vi "Loop_SM.vi"() -> ()   [LabVIEW 2017, in "Claw_Rotation.lvlib"]
uses:
  Claw_Rotation.lvlib
  CLUSTER_CMD_SM_Lift_Rotate.ctl
  ENUM_SM_Rotate_Positions.ctl
  _SHARE ALL/TypeDef Share All/CLUSTER_TalonInput.ctl
  System Drivers/Phoenix-LabVIEW/Motor Controller/Controls/CTRE_Phoenix_MotorControl_ControlMode.ctl
  TypeDef/CLUSTER_PID.ctl
  ENUM_SM_State.ctl
  CLUSTER_ACT_Lift Output.ctl
  _SHARE ALL/RoboRio Share All/SRX Share All/TypeDefs SRX/Cluster_SRX_General Data.ctl
  _SHARE ALL/RoboRio Share All/SRX Share All/TypeDefs SRX/Cluster_SRX_Common Runtime Data.ctl
  _SHARE ALL/RoboRio Share All/SRX Share All/TypeDefs SRX/Cluster_SRX_Error Calculations.ctl
  _SHARE ALL/RoboRio Share All/SRX Share All/TypeDefs SRX/Cluster_SRX_Voltage Out Data.ctl
  _SHARE ALL/RoboRio Share All/SRX Share All/TypeDefs SRX/Cluster_SRX_Sensor Out Data.ctl
  _SHARE ALL/RoboRio Share All/SRX Share All/TypeDefs SRX/Cluster_SRX_Sensor Quad Data.ctl
  _SHARE ALL/RoboRio Share All/SRX Share All/TypeDefs SRX/Cluster_SRX_Analog In Data.ctl
  _SHARE ALL/RoboRio Share All/SRX Share All/TypeDefs SRX/Cluster_SRX_PWM Sensor Data.ctl
  _SHARE ALL/RoboRio Share All/SRX Share All/TypeDefs SRX/Cluster_SRX_F and R Limit Indicators.ctl
  ENUM_SM_Action.ctl
  Globals/Global_Device_IDs.vi
  _SHARE ALL/Global Share All/Global_STOP.vi
  Global_ACT Write_Data Out.vi
  Global_SM Write_Data Out.vi
  Global_CMD.vi
panel:
  in  "CMD_SM_Claw_Rotation":T1={"Enable System"=TRUE, "Rotate Position"=enum."Neutral: 0", "Manual Velocity"=0.0, "Manual Mode"=FALSE}
  out "State":T3
  out "SM Output":T4 {"Talon Mode" items=["PercentOutput"=0, "Position"=1, "Velocity"=2, "Current"=3, "Follower"=5, "MotionProfile"=6, "MotionMagic"=7, "MotionMagicArc"=8, "MotionProfileArc"=10, "Disabled"=15]}
  out "SM CMD Input":T1={"Enable System"=TRUE, "Rotate Position"=enum."Neutral: 0", "Manual Velocity"=0.0, "Manual Mode"=FALSE}
  out "Cycle Time (S)":dbl format="%.3g"
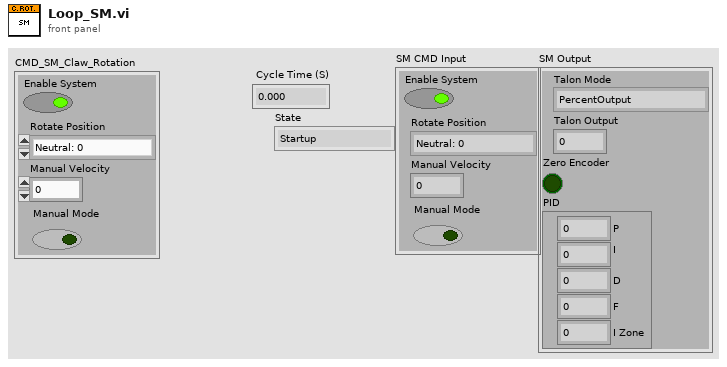
[diagram p1: front panel]
types:
  T1 = typedef "Claw_Rotation.lvlib/CLUSTER_CMD_SM_Lift_Rotate.ctl" = cluster{"Enable System":bool, "Rotate Position":T2, "Manual Velocity":dbl, "Manual Mode":bool}
  T2 = typedef "Claw_Rotation.lvlib/ENUM_SM_Rotate_Positions.ctl" = enum16{"Neutral: 0", "Pickup: 0", "Exchange: 0", "Switch: 0", "Scale: 0", "Climb: 0"}
  T3 = typedef "Claw_Rotation.lvlib/ENUM_SM_State.ctl" = enum16{"Startup", "Idle", "Manual", "Position - Moving", "Position - Holding", "Shutdown"}
  T4 = typedef "CLUSTER_TalonInput.ctl" = cluster{"Talon Mode":T5, "Talon Output":dbl, "Zero Encoder":bool, "PID":T6}
  T5 = typedef "CTRE_Phoenix_MotorControl_ControlMode.ctl" = u16
  T6 = typedef "CLUSTER_PID.ctl" = cluster{"P":dbl, "I":dbl, "D":dbl, "F":dbl, "I Zone":dbl}
  T7 = typedef "Claw_Rotation.lvlib/CLUSTER_ACT_Lift Output.ctl" = cluster{"Device Info Out":T8, "Common Runtime Data Out":T9, "Quad Sensor Data Out":T13, "Analog Sensor Data Out":T14, "PWM Data Out":T15, "Hard Limits Out":T16}
  T8 = typedef "Cluster_SRX_General Data.ctl" = cluster{"Device ID":i32, "Firmware Version":i32, "Inverted?":bool, "Has Reset Occurred?":bool}
  T9 = typedef "Cluster_SRX_Common Runtime Data.ctl" = cluster{"Calc":T10, "Voltage ":T11, "Sensor":T12, "Current":dbl, "Temp":dbl}
  T10 = typedef "Cluster_SRX_Error Calculations.ctl" = cluster{"Error":i32, "D-Error":dbl, "I-Acc":dbl}
  T11 = typedef "Cluster_SRX_Voltage Out Data.ctl" = cluster{"Percent":dbl, "Output":dbl, "Bus":dbl}
  T12 = typedef "Cluster_SRX_Sensor Out Data.ctl" = cluster{"Pos":i32, "Vel":i32}
  T13 = typedef "Cluster_SRX_Sensor Quad Data.ctl" = cluster{"Position":i32, "Velocity":i32, "Quad A Pin":bool, "Quad B Pin":bool, "Quad Idx Pin":bool}
  T14 = typedef "Cluster_SRX_Analog In Data.ctl" = cluster{"WithOv":i32, "Raw":i32, "Velocity":i32}
  T15 = typedef "Cluster_SRX_PWM Sensor Data.ctl" = cluster{"Position":i32, "Velocity":i32, "High(us)":i32, "Period(us)":i32}
  T16 = typedef "Cluster_SRX_F and R Limit Indicators.ctl" = cluster{"Forward Closed?":bool, "Reverse Closed?":bool}
  T17 = typedef "Claw_Rotation.lvlib/ENUM_SM_Action.ctl" = enum16{"No Action", "Reset Time", "Reset All", "Reset Encoder", "Manual", "Position", "Set PID 1", "Disable Motor"}
  T18 = typedef "CLUSTER_Talon_Setup.ctl" = cluster{"Open Data":T19, "Current Config Data":T20, "Sensor Config":T21, "Hard Limits":T23, "Motion Magic Config Data":T25, "PIDF":T26, "Maximum Integral Accumulator Value":dbl, "AllowableClosedLoop":i32, "Limits":T27, "Output Config":T28}
  T19 = typedef "Cluster_SRX_OPEN Data.ctl" = cluster{"SRX ID":u8, "Invert Output":bool}
  T20 = typedef "Cluster_SRX_Current Config.ctl" = cluster{"Enable Current Limit?":bool, "Peak Current (Amps)":i32, "Peak Current Maximum Duration (ms)":i32, "Continuous Current Limit (Amps)":i32}
  T21 = typedef "Cluster_SRX_Sensor Config.ctl" = cluster{"Feedback Device":T22, "PhaseSensor":bool}
  T22 = typedef "CTRE_Phoenix_MotorControl_FeedbackDevice.ctl" = i8
  T23 = typedef "Cluster_SRX_Config Hard Limits.ctl" = cluster{"Fwd Enable":bool, "Rev Enable":bool, "Fwd NO-NC":T24, "Rev NO-NC":T24}
  T24 = typedef "CTRE_Phoenix_MotorControl_LimitSwitchNormal.ctl" = enum16{"Normally Open", "Normally Closed", "Disabled"}
  T25 = typedef "Cluster_SRX_Motion Magic Config Data.ctl" = cluster{"Cruise Velocity":i32, "Acceleration":i32}
  T26 = typedef "Cluster_SRX_PIDF.ctl" = cluster{"P":dbl, "I":dbl, "D":dbl, "F":dbl, "I Zone":dbl}
  T27 = typedef "Cluster_SRX_Config Soft Limits.ctl" = cluster{"Max":i32, "Min":i32, "Max Enable":bool, "Min Enable":bool}
  T28 = typedef "Cluster_SRX_Config Voltage Output.ctl" = cluster{"Invert?":bool, "Neutral Mode":T29, "Deadband (-1to1)":dbl, "Ramp Time Off to Full (S)":dbl, "Peak  (-1to1)":T30, "Nominal  (-1to1)":T30}
  T29 = typedef "CTRE_Phoenix_MotorControl_NeutralMode.ctl" = enum8{"EEPROMSetting", "Override to Coast", "Override to Brake"}
  T30 = typedef "Cluster_SRX_Forward and Reverse.ctl" = cluster{"Forward":dbl, "Reverse":dbl}
  T31 = cluster{"State":T3, "Previous State":T3, "Current Time":timestamp, "Previous Time":timestamp, "Start Time":timestamp, "Target Time (ms)":u32, "Cycle Time(S)":dbl, "Claw_Rotation_Output":T7, "SM CMD Input":T1, "SM Output":T4, "Claw Rotation Setup":T18}
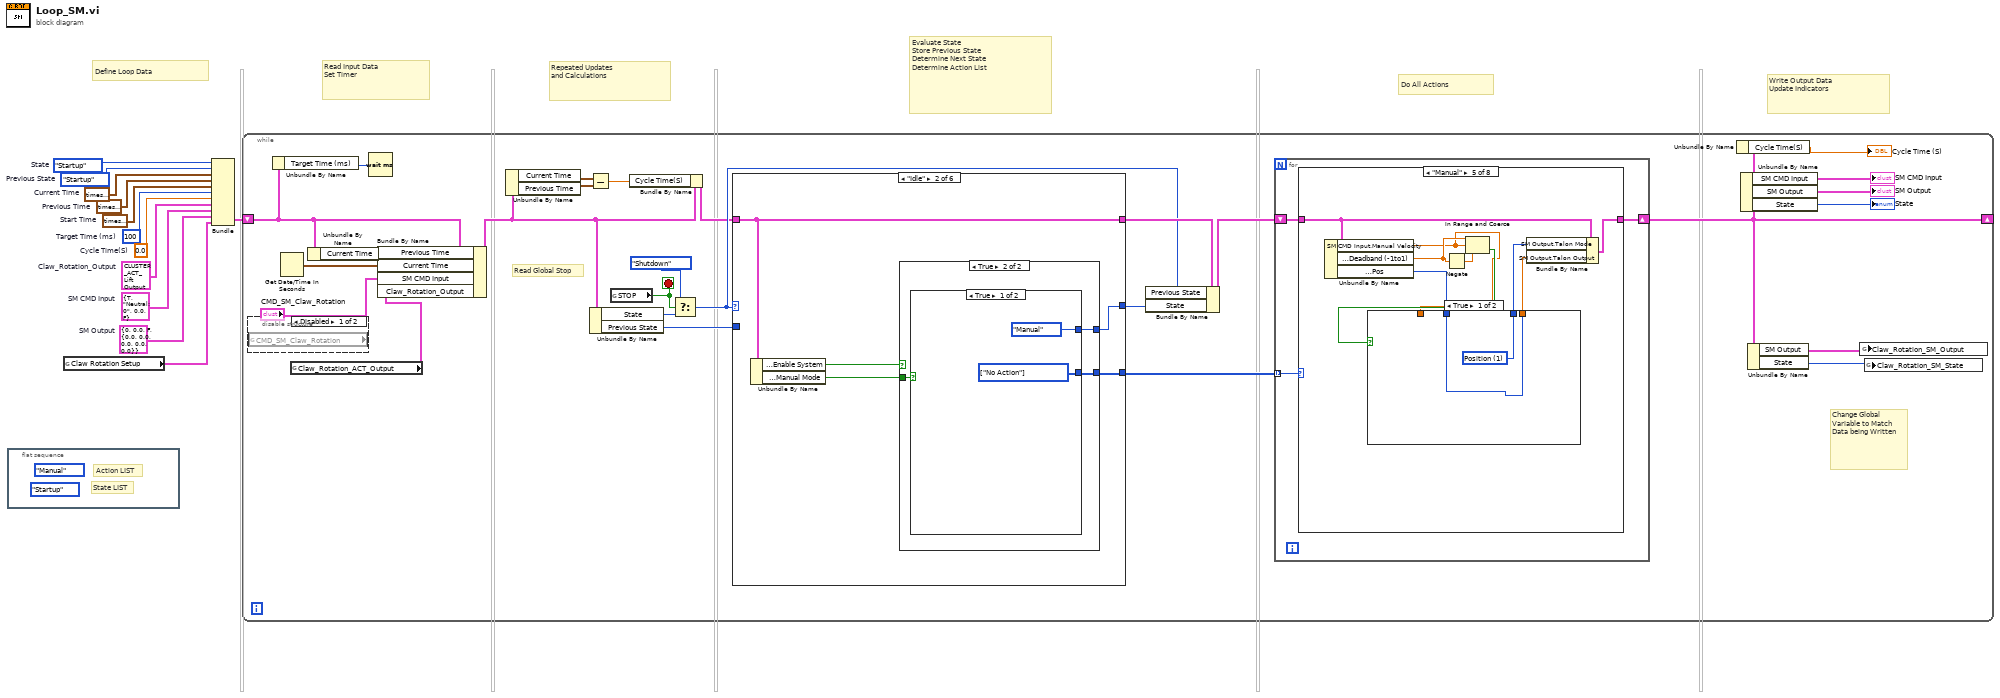
[diagram p0: block diagram]
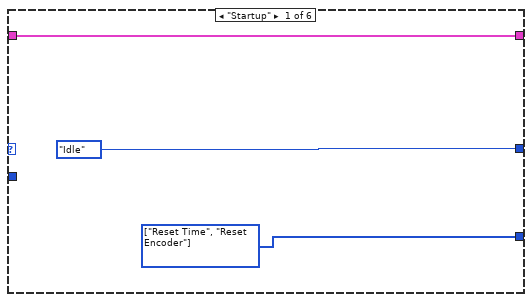
[diagram p3: hidden frame]
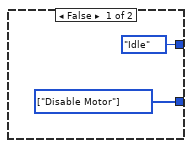
[diagram p4: hidden frame]
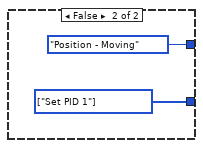
[diagram p5: hidden frame]
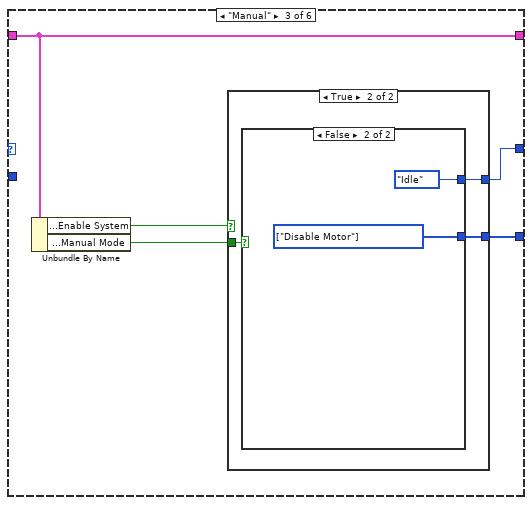
[diagram p6: hidden frame]
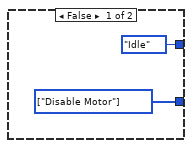
[diagram p7: hidden frame]
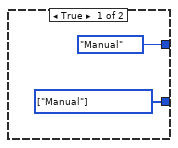
[diagram p8: hidden frame]
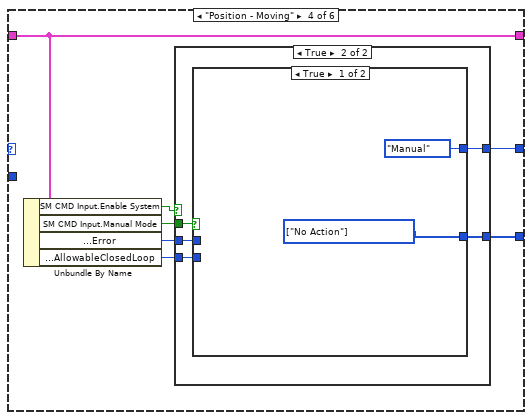
[diagram p9: hidden frame]
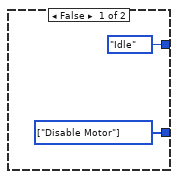
[diagram p10: hidden frame]
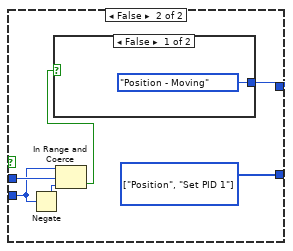
[diagram p11: hidden frame]
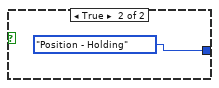
[diagram p12: hidden frame]
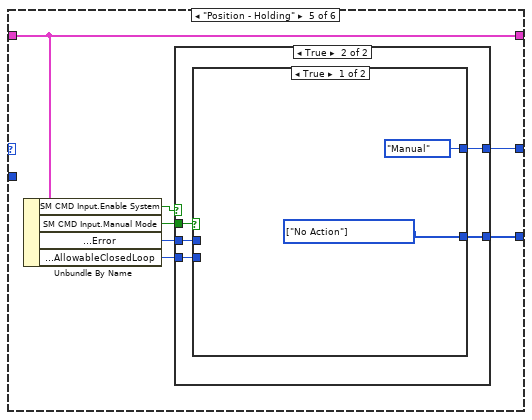
[diagram p13: hidden frame]
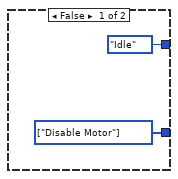
[diagram p14: hidden frame]
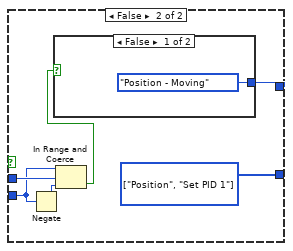
[diagram p15: hidden frame]
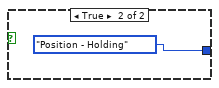
[diagram p16: hidden frame]
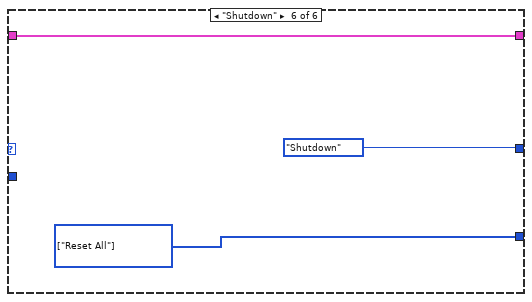
[diagram p17: hidden frame]
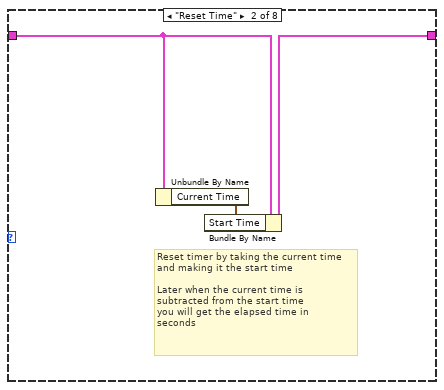
[diagram p19: hidden frame]
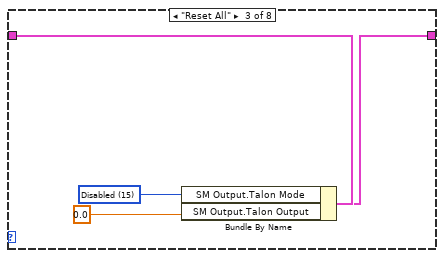
[diagram p20: hidden frame]
diagram:
  w2 = T4 {"Talon Mode"=0, "Talon Output"=0.0, "Zero Encoder"=FALSE, "PID"={"P"=0.0, "I"=0.0, "D"=0.0, "F"=0.0, "I Zone"=0.0}}  # SM Output
  w3 = T1 {"Enable System"=TRUE, "Rotate Position"=enum."Neutral: 0", "Manual Velocity"=0.0, "Manual Mode"=FALSE}  # SM CMD Input
  w4 = T7 {"Device Info Out"={"Device ID"=0, "Firmware Version"=0, "Inverted?"=FALSE, "Has Reset Occurred?"=FALSE}, "Common Runtime Data Out"={"Calc"={"Error"=0, "D-Error"=0.0, "I-Acc"=0.0}, "Voltage "={"Percent"=0.0, "Output"=0.0, "Bus"=0.0}, "Sensor"={"Pos"=0, "Vel"=0}, "Current"=0.0, "Temp"=0.0}, "Quad Sensor Data Out"={"Position"=0, "Velocity"=0, "Quad A Pin"=FALSE, "Quad B Pin"=FALSE, "Quad Idx Pin"=FALSE}, "Analog Sensor Data Out"={"WithOv"=0, "Raw"=0, "Velocity"=0}, "PWM Data Out"={"Position"=0, "Velocity"=0, "High(us)"=0, "Period(us)"=0}, "Hard Limits Out"={"Forward Closed?"=FALSE, "Reverse Closed?"=FALSE}}  # Claw_Rotation_Output
  w5 = 0.0  # Cycle Time(S)
  w6 = ENUM_SM_State."Startup"  # Previous State
  w7 = timestamp(0 s since 1904-01-01)  # Previous Time
  w8 = u32 100  # Target Time (ms)
  w9 = timestamp(0 s since 1904-01-01)  # Start Time
  w10 = timestamp(0 s since 1904-01-01)  # Current Time
  w11 = ENUM_SM_State."Startup"  # State
  # "Define Loop Data"
  # "Repeated Updates\nand Calculations"
  # "Read Input Data\nSet Timer"
  # "Evaluate State\nStore Previous State\nDetermine Next State\nDetermine Action List"
  # "Do All Actions"
  # "Write Output Data\nUpdate Indicators"
  n1 = flat-sequence {
    frame #0 {
      (unwired) ENUM_SM_State."Startup" ("State")
      (unwired) ENUM_SM_Action."Manual" ("Action")
      # "State LIST"
      # "Action LIST"
    }
  }
  n2 = global read "Global_Device_IDs.vi" "Claw Rotation Setup"() -> (w1:T18)
  n3 = Bundle("State"=w11, "Previous State"=w6, "Current Time"=w10, "Previous Time"=w7, "Start Time"=w9, "Target Time (ms)"=w8, "Cycle Time(S)"=w5, "Claw_Rotation_Output"=w4, "SM CMD Input"=w3, "SM Output"=w2, "Claw Rotation Setup"=w1) -> (w12:T31)  [unwired: 1 in]
  n4 = while {
    shift-right: [w28] -> _
    shift-left: w12 -> [w31]
    stop <- w36 stop-if-true
    # "Change Global\nVariable to Match\nData being Written"
    # "Read Global Stop"
    n5 = disable-structure shown="Disabled" {
      frame Disabled {
        n6 = global read "Global_CMD.vi" "CMD_SM_Claw_Rotation"() -> (w40:T1)
      }
      frame Enabled {
      }
    }
    n7 = Unbundle By Name(w31) -> ("Target Time (ms)"=w33:u32)
    n8 = Get Date/Time In Seconds() -> (seconds since 1Jan1904=w39:timestamp)
    n9 = global read "Global_ACT Write_Data Out.vi" "Claw_Rotation_ACT_Output"() -> (w20:T7)
    n10 = Unbundle By Name(w31) -> ("Current Time"=w32:timestamp)
    n11 = Wait (ms)(milliseconds to wait=w33) -> ()  [unwired: 1 out]
    n12 = Bundle By Name(cluster=w31, "Previous Time"=w32, "Current Time"=w39, "SM CMD Input"="CMD_SM_Claw_Rotation", "Claw_Rotation_Output"=w20) -> (w24:T31)
    n13 = Unbundle By Name(w24) -> ("Current Time"=w25:timestamp, "Previous Time"=w26:timestamp)
    n14 = Subtract(x=w25, y=w26) -> (x-y=w22:dbl)
    n15 = Unbundle By Name(w24) -> ("State"=w34:T3, "Previous State"=w30:T3)
    n16 = global read "Global_STOP.vi" "STOP"() -> (w36:bool)
    n17 = Bundle By Name(cluster=w24, "Cycle Time(S)"=w22) -> (w23:T31)
    n18 = Select(t=ENUM_SM_State."Shutdown" ("State"), s=w36, f=w34) -> (s? t:f=w29:T3)
    n19 = case shown="\"Idle\"" w29 {
      tunnel: w23 -> [w43 w48 w62 w78 w102 w122]
      tunnel: [w43 w48 w62 w78 w102 w122] -> w37
      tunnel: [w42 w44 w58 w74 w98 w121] -> w21
      tunnel: w30 -> [_ _ _ _ _ _]
      tunnel: [ENUM_SM_State."Idle" ("State") w45 w59 w73 w97 ENUM_SM_State."Shutdown" ("State")] -> w19
      frame "Startup" {
        w42 = T17[] [enum."Reset Time", enum."Reset Encoder"] items=["No Action", "Reset Time", "Reset All", "Reset Encoder", "Manual", "Position", "Set PID 1", "Disable Motor"] ("Actions")
      }
      frame "Idle" {
        n20 = Unbundle By Name(w48) -> ("SM CMD Input.Enable System"=w47:bool, "SM CMD Input.Manual Mode"=w46:bool)
        n21 = case shown="True" w47 {
          tunnel: w46 -> [_ w53]
          tunnel: [ENUM_SM_State."Idle" ("State") w52] -> w45
          tunnel: [w49 w51] -> w44
          frame False {
            w49 = T17[] [enum."Disable Motor"] items=["No Action", "Reset Time", "Reset All", "Reset Encoder", "Manual", "Position", "Set PID 1", "Disable Motor"] ("Actions")
          }
          frame True {
            n22 = case shown="True" w53 {
              tunnel: [ENUM_SM_State."Manual" ("State") ENUM_SM_State."Position - Moving" ("State")] -> w52
              tunnel: [w54 w56] -> w51
              frame True {
                w54 = T17[] [enum."No Action"] items=["No Action", "Reset Time", "Reset All", "Reset Encoder", "Manual", "Position", "Set PID 1", "Disable Motor"] ("Actions")
              }
              frame False {
                w56 = T17[] [enum."Set PID 1"] items=["No Action", "Reset Time", "Reset All", "Reset Encoder", "Manual", "Position", "Set PID 1", "Disable Motor"] ("Actions")
              }
            }
          }
        }
      }
      frame "Manual" {
        n23 = Unbundle By Name(w62) -> ("SM CMD Input.Enable System"=w61:bool, "SM CMD Input.Manual Mode"=w60:bool)
        n24 = case shown="True" w61 {
          tunnel: w60 -> [_ w67]
          tunnel: [ENUM_SM_State."Idle" ("State") w66] -> w59
          tunnel: [w63 w65] -> w58
          frame False {
            w63 = T17[] [enum."Disable Motor"] items=["No Action", "Reset Time", "Reset All", "Reset Encoder", "Manual", "Position", "Set PID 1", "Disable Motor"] ("Actions")
          }
          frame True {
            n25 = case shown="False" w67 {
              tunnel: [ENUM_SM_State."Manual" ("State") ENUM_SM_State."Idle" ("State")] -> w66
              tunnel: [w68 w70] -> w65
              frame True {
                w68 = T17[] [enum."Manual"] items=["No Action", "Reset Time", "Reset All", "Reset Encoder", "Manual", "Position", "Set PID 1", "Disable Motor"] ("Actions")
              }
              frame False {
                w70 = T17[] [enum."Disable Motor"] items=["No Action", "Reset Time", "Reset All", "Reset Encoder", "Manual", "Position", "Set PID 1", "Disable Motor"] ("Actions")
              }
            }
          }
        }
      }
      frame "Position - Moving" {
        n26 = Unbundle By Name(w78) -> ("SM CMD Input.Enable System"=w72:bool, "SM CMD Input.Manual Mode"=w77:bool, "Claw_Rotation_Output.Common Runtime Data Out.Calc.Error"=w76:i32, "Claw Rotation Setup.AllowableClosedLoop"=w75:i32)
        n27 = case shown="True" w72 {
          tunnel: w77 -> [_ w85]
          tunnel: w76 -> [_ w84]
          tunnel: w75 -> [_ w83]
          tunnel: [w79 w82] -> w74
          tunnel: [ENUM_SM_State."Idle" ("State") w81] -> w73
          frame False {
            w79 = T17[] [enum."Disable Motor"] items=["No Action", "Reset Time", "Reset All", "Reset Encoder", "Manual", "Position", "Set PID 1", "Disable Motor"] ("Actions")
          }
          frame True {
            n28 = case shown="True" w85 {
              tunnel: w84 -> [_ w93]
              tunnel: w83 -> [_ w92]
              tunnel: [w86 w89] -> w82
              tunnel: [ENUM_SM_State."Manual" ("State") w88] -> w81
              frame True {
                w86 = T17[] [enum."No Action"] items=["No Action", "Reset Time", "Reset All", "Reset Encoder", "Manual", "Position", "Set PID 1", "Disable Motor"] ("Actions")
              }
              frame False {
                w89 = T17[] [enum."Position", enum."Set PID 1"] items=["No Action", "Reset Time", "Reset All", "Reset Encoder", "Manual", "Position", "Set PID 1", "Disable Motor"] ("Actions")
                n29 = Negate(x=w92) -> (-x=w91:i32)
                n30 = In Range and Coerce(upper limit=w92, x=w93, lower limit=w91) -> (In Range?=w90:bool)  [unwired: 1 out]
                n31 = case shown="False" w90 {
                  tunnel: [ENUM_SM_State."Position - Moving" ("State") ENUM_SM_State."Position - Holding" ("State")] -> w88
                  frame False {
                  }
                  frame True {
                  }
                }
              }
            }
          }
        }
      }
      frame "Position - Holding" {
        n32 = Unbundle By Name(w102) -> ("SM CMD Input.Enable System"=w96:bool, "SM CMD Input.Manual Mode"=w101:bool, "Claw_Rotation_Output.Common Runtime Data Out.Calc.Error"=w100:i32, "Claw Rotation Setup.AllowableClosedLoop"=w99:i32)
        n33 = case shown="True" w96 {
          tunnel: w101 -> [_ w109]
          tunnel: w100 -> [_ w108]
          tunnel: w99 -> [_ w107]
          tunnel: [w103 w106] -> w98
          tunnel: [ENUM_SM_State."Idle" ("State") w105] -> w97
          frame False {
            w103 = T17[] [enum."Disable Motor"] items=["No Action", "Reset Time", "Reset All", "Reset Encoder", "Manual", "Position", "Set PID 1", "Disable Motor"] ("Actions")
          }
          frame True {
            n34 = case shown="True" w109 {
              tunnel: w108 -> [_ w117]
              tunnel: w107 -> [_ w116]
              tunnel: [w110 w113] -> w106
              tunnel: [ENUM_SM_State."Manual" ("State") w112] -> w105
              frame True {
                w110 = T17[] [enum."No Action"] items=["No Action", "Reset Time", "Reset All", "Reset Encoder", "Manual", "Position", "Set PID 1", "Disable Motor"] ("Actions")
              }
              frame False {
                w113 = T17[] [enum."Position", enum."Set PID 1"] items=["No Action", "Reset Time", "Reset All", "Reset Encoder", "Manual", "Position", "Set PID 1", "Disable Motor"] ("Actions")
                n35 = Negate(x=w116) -> (-x=w115:i32)
                n36 = In Range and Coerce(upper limit=w116, x=w117, lower limit=w115) -> (In Range?=w114:bool)  [unwired: 1 out]
                n37 = case shown="False" w114 {
                  tunnel: [ENUM_SM_State."Position - Moving" ("State") ENUM_SM_State."Position - Holding" ("State")] -> w112
                  frame False {
                  }
                  frame True {
                  }
                }
              }
            }
          }
        }
      }
      frame "Shutdown" {
        w121 = T17[] [enum."Reset All"] items=["No Action", "Reset Time", "Reset All", "Reset Encoder", "Manual", "Position", "Set PID 1", "Disable Motor"] ("Actions")
      }
    }
    n38 = Bundle By Name(cluster=w37, "Previous State"=w29, "State"=w19) -> (w38:T31)
    n39 = for {
      tunnel: w21 -> [w125] mode=indexing
      shift-right: [w124] -> w28
      shift-left: w38 -> [w123]
      n40 = case shown="\"Manual\"" w125 {
        tunnel: w123 -> [w126 w129 w133 w136 w142 w157 w160 w164]
        tunnel: [w126 w128 w132 w135 w141 w158 w161 w163] -> w124
        frame "No Action" {
        }
        frame "Reset Time" {
          # "Reset timer by taking the current time\nand making it the start time\n\nLater when the current time is \nsubtracted from the start time\nyou will get the elapsed time in \nseconds"
          n41 = Unbundle By Name(w129) -> ("Current Time"=w127:timestamp)
          n42 = Bundle By Name(cluster=w129, "Start Time"=w127) -> (w128:T31)
        }
        frame "Reset All" {
          w131 = T5 15 items=["PercentOutput"=0, "Position"=1, "Velocity"=2, "Current"=3, "Follower"=5, "MotionProfile"=6, "MotionMagic"=7, "MotionMagicArc"=8, "MotionProfileArc"=10, "Disabled"=15] ("SM Output.Talon Mode")
          n43 = Bundle By Name(cluster=w133, "SM Output.Talon Mode"=w131, "SM Output.Talon Output"=0.0) -> (w132:T31)
        }
        frame "Reset Encoder" {
          n44 = Bundle By Name(cluster=w136, "SM Output.Zero Encoder"=TRUE) -> (w135:T31)
        }
        frame "Manual" {
          n45 = Unbundle By Name(w142) -> ("SM CMD Input.Manual Velocity"=w140:dbl, "Claw Rotation Setup.Output Config.Deadband (-1to1)"=w145:dbl, "Claw_Rotation_Output.Common Runtime Data Out.Sensor.Pos"=w137:i32)
          n46 = Negate(x=w145) -> (-x=w144:dbl)
          n47 = In Range and Coerce(upper limit=w145, x=w140, lower limit=w144) -> (In Range?=w143:bool)  [unwired: 1 out]
          n48 = case shown="True" w143 {
            tunnel: w140 -> [_ w148]
            tunnel: [w147 w149] -> w139
            tunnel: [w146 w148] -> w138
            tunnel: w137 -> [w146 _]
            frame True {
              w147 = T5 1 items=["PercentOutput"=0, "Position"=1, "Velocity"=2, "Current"=3, "Follower"=5, "MotionProfile"=6, "MotionMagic"=7, "MotionMagicArc"=8, "MotionProfileArc"=10, "Disabled"=15] ("SM Output.Talon Mode")
            }
            frame False {
              w149 = T5 0 items=["PercentOutput"=0, "Position"=1, "Velocity"=2, "Current"=3, "Follower"=5, "MotionProfile"=6, "MotionMagic"=7, "MotionMagicArc"=8, "MotionProfileArc"=10, "Disabled"=15] ("SM Output.Talon Mode")
            }
          }
          n49 = Bundle By Name(cluster=w142, "SM Output.Talon Mode"=w139, "SM Output.Talon Output"=w138) -> (w141:T31)
        }
        frame "Position" {
          n50 = Unbundle By Name(w157) -> ("SM CMD Input.Rotate Position"=w151:T2)
          n51 = Format Into String(w151) -> (resulting string=w156:string)  [unwired: 3 in, 1 out]
          n52 = Match Pattern(string=w156, regular expression=":") -> (before substring=w154:string, after substring=w153:string)  [unwired: 1 in, 2 out]
          n53 = call <vilib>:"Trim Whitespace.vi"("string"=w154) -> ()  [unwired: 1 in, 1 out]
          n54 = call <vilib>:"Trim Whitespace.vi"("string"=w153) -> ("trimmed string"=w152:string)  [unwired: 1 in]
          n55 = Decimal String To Number(string=w152) -> (number=w150:i32)  [unwired: 2 in, 1 out]
          n56 = Bundle By Name(cluster=w157, "SM Output.Talon Output"=w150) -> (w158:T31)
        }
        frame "Set PID 1" {
          n57 = Unbundle By Name(w160) -> ("Claw Rotation Setup.PIDF"=w159:T26)
          n58 = Bundle By Name(cluster=w160, "SM Output.PID"=w159) -> (w161:T31)
        }
        frame "Disable Motor" {
          w162 = T5 15 items=["PercentOutput"=0, "Position"=1, "Velocity"=2, "Current"=3, "Follower"=5, "MotionProfile"=6, "MotionMagic"=7, "MotionMagicArc"=8, "MotionProfileArc"=10, "Disabled"=15] ("SM Output.Talon Mode")
          n59 = Bundle By Name(cluster=w164, "SM Output.Talon Mode"=w162) -> (w163:T31)
        }
      }
    }
    n60 = Unbundle By Name(w28) -> ("Cycle Time(S)"=→"Cycle Time (S)":dbl)
    n61 = Unbundle By Name(w28) -> ("SM CMD Input"=→"SM CMD Input":T1, "SM Output"=→"SM Output":T4, "State"=→"State":T3)
    n62 = Unbundle By Name(w28) -> ("SM Output"=w17:T4, "State"=w18:T3)
    n63 = global write "Global_SM Write_Data Out.vi" "Claw_Rotation_SM_Output"(w17) -> ()
    n64 = global write "Global_SM Write_Data Out.vi" "Claw_Rotation_SM_State"(w18) -> ()
  }
